vi "Read TuningParameters.vi"(8 "error in (no error)":errorcluster, 11 "BuckBoost configuration in":refnum<class "BuckBoost configuration.lvclass">) -> (0 "error out":errorcluster, 2 "TuningParameters":T1 {"gains"."proportional gain" step=0.125}, 3 "BuckBoost configuration out":refnum<class "BuckBoost configuration.lvclass">)   [LabVIEW 2017, in "BuckBoost configuration.lvclass"]
uses:
  BuckBoost configuration.lvclass
  <vilib>/NI/PowerElectronicsControl/Buck-Boost/RealTime/TuningParameters.ctl
  <vilib>/rvi/Analysis/control/PID/Typedef/niFpgaPID_PIGains.ctl
  <vilib>/NI/PowerElectronicsControl/Buck-Boost/FPGA/contState.ctl
  BuckBoost configuration.lvclass/BuckBoost configuration.ctl
  <vilib>/NI/PowerElectronicsControl/Buck-Boost/FPGA/BuckBoost.lvlib
  <vilib>/NI/PowerElectronicsControl/Buck-Boost/RealTime/BuckBoostInterface.lvlib
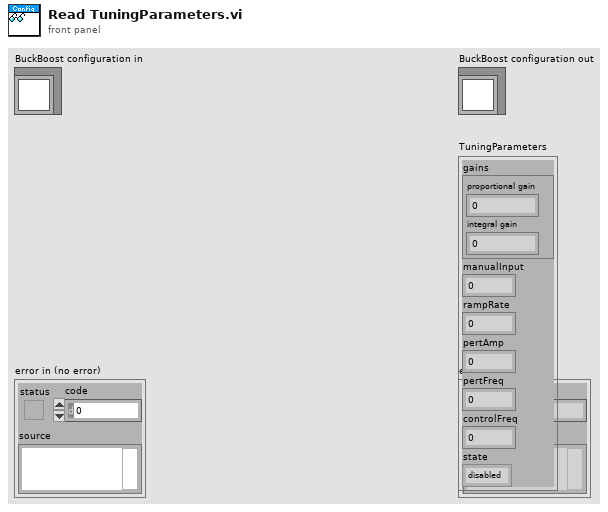
[diagram p1: front panel]
types:
  T1 = typedef "BuckBoostInterface.lvlib/TuningParameters.ctl" = cluster{"gains":T2, "manualInput":sgl, "rampRate":sgl, "pertAmp":sgl, "pertFreq":sgl, "controlFreq":sgl, "state":T3}
  T2 = typedef "niFpgaPID_PIGains.ctl" = cluster{"proportional gain":sgl, "integral gain":sgl}
  T3 = typedef "BuckBoost.lvlib/contState.ctl" = enum16{"disabled", "manual", "normal", "perturb"}
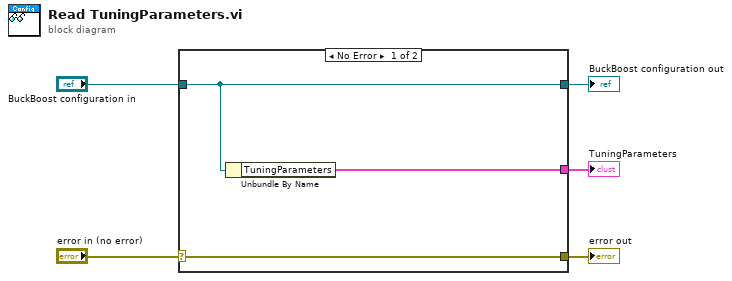
[diagram p0: block diagram]
diagram:
  n1 = case shown="No Error" "error in (no error)" {
    selector: "error in (no error)" -> [w8 w9]
    tunnel: [w8 w9] -> w4
    tunnel: [w7 w10] -> w2
    tunnel: "BuckBoost configuration in" -> [w7 w10]
    tunnel: [w6 _] -> w1
    frame No Error {
      n2 = Unbundle By Name(w7) -> ("TuningParameters"=w6:T1)
    }
    frame Error {
    }
  }
  "error out" <- w4
  "BuckBoost configuration out" <- w2
  "TuningParameters" <- w1
